vi "User Actor Core Close.vi"(0 "Module in":refnum<class "Module.lvclass">, 11 "Error in":errorcluster caption="Error in (no error)") -> (4 "Module out":refnum<class "Module.lvclass">, 15 "Error out":errorcluster)   [LabVIEW 2019, in "GP Module.lvlib" / "Module.lvclass"]
doc: "Close custom resources opened during <B>Actor</B> initialization or run. Typical actions:\n\n- Close own references.\n- Deinitialize SW resources.\n- Deinitialize HW resources.\n- Unregister or destroy additional user events.\n\n<B>You should not invoke the Call Parent Method node when adding this override.</B>\n\nDefault action\n---------------\nNo action.\n\nSteen Schmidt\nGPower\n8/5 2017"
uses:
  Module.lvclass
  C:/Program Files (x86)/National Instruments/LabVIEW 2019/vi.lib/GPower/Actor/Library/Actor Class/Actor.lvclass
  <vilib>/GPower/Actor/Library/Actor Class/Actor.lvclass/Actor.ctl
  <vilib>/GPower/Actor/Library/Actor Interface Class/Actor Interface.lvclass/Actor Interface.ctl
  <vilib>/GPower/Actor/Library/Actor Class/Actor.lvclass
  <vilib>/GPower/UI/Library/GP UI.lvlib
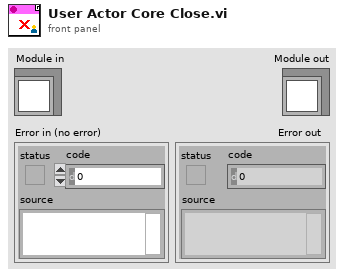
[diagram p1: front panel]
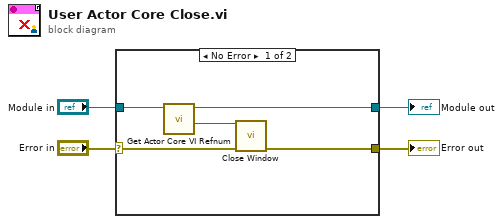
[diagram p0: block diagram]
diagram:
  n1 = case shown="No Error" "Error in" {
    selector: "Error in" -> [w7 w11]
    tunnel: [w6 w11] -> w3
    tunnel: "Module in" -> [w9 w10]
    tunnel: [w8 w10] -> w1
    frame No Error {
      n2 = call <vilib>:"Get Actor Core VI Refnum.vi"("Actor in"=w9) -> ("Actor Core VI Refnum"=w5:refnum<vi>, "Actor out"=w8:refnum<class "Module.lvclass">)  [unwired: 9 in]
      n3 = call <vilib>:"Close Window.vi"("VI Refnum"=w5, "Error in"=w7) -> ("Error out"=w6:errorcluster)  [unwired: 13 in]
    }
    frame Error {
    }
  }
  "Module out" <- w1
  "Error out" <- w3
